vi "Create Buffer.vi"(6 "error in (no error)":errorcluster, 9 "Driver":refnum<class "Driver.lvclass">) -> (0 "error out":errorcluster, 3 "CommandDirector":refnum<class "CommandDirector.lvclass">)   [LabVIEW 2023]
uses:
  User Defined Write/User Defined Write.lvclass
  CommandDirector/CommandDirector.lvclass
  \\Mac\Home/Documents/LabVIEW Data/ProjectTemplates/Source/HAF/WriteCommand/WriteCommand.lvclass
  \\Mac\Home/Documents/LabVIEW Data/ProjectTemplates/Source/HAF/Executable/Executable.lvclass
  \\Mac\Home/Documents/LabVIEW Data/ProjectTemplates/Source/HAF/User Defined Write/User Defined Write.lvclass
  Driver/Driver.lvclass
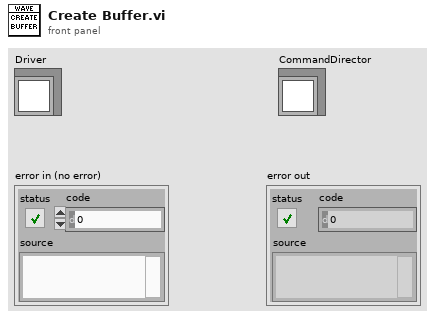
[diagram p1: front panel]
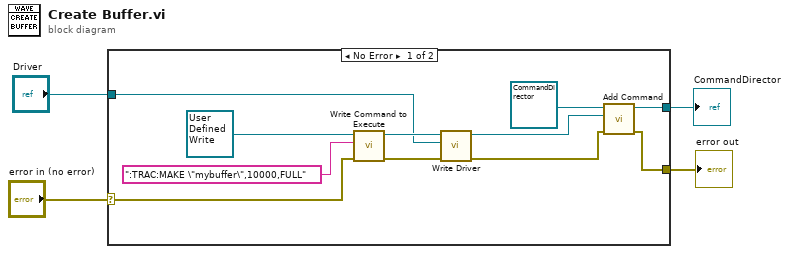
[diagram p0: block diagram]
diagram:
  n1 = case shown="No Error" "error in (no error)" {
    selector: "error in (no error)" -> [w13 w16]
    tunnel: "Driver" -> [w11 _]
    tunnel: [w6 _] -> w2
    tunnel: [w5 w16] -> w1
    frame No Error {
      n2 = call-dynamic "Write Command to Execute.vi"("error in (no error)"=w13, "Command to Execute"=":TRAC:MAKE \"mybuffer\",10000,FULL", "User Defined Write in"=refnum<class "User Defined Write.lvclass"> refnum ("HAF:User Defined Write.lvclass")) -> ("error out"=w10:errorcluster, "User Defined Write out"=w12:refnum<class "User Defined Write.lvclass">)  [unwired: 7 in]
      n3 = call-dynamic "Write Driver.vi"("error in (no error)"=w10, "HAF:Driver.lvclass"=w11, "WriteCommand in"=w12) -> ("error out"=w7:errorcluster, "WriteCommand out"=w8:refnum<class "User Defined Write.lvclass">)  [unwired: 7 in]
      n4 = call-dynamic "Add Command.vi"("error in (no error)"=w7, "Write Command"=w8, "Command Director in"=refnum<class "CommandDirector.lvclass"> refnum ("HAF:CommandDirector.lvclass")) -> ("error out"=w5:errorcluster, "Command Director out"=w6:refnum<class "CommandDirector.lvclass">)  [unwired: 7 in]
    }
    frame Error {
    }
  }
  "error out" <- w1
  "CommandDirector" <- w2
